vi "SetAllOccurrences.vi"(0 "occurrences":refnum<k4>[](array[refnum])) -> ()   [LabVIEW 2019, in "MessengerM.lvlib" / "SubChannelCPU.lvclass"]
uses:
  SubChannelCPU.lvclass
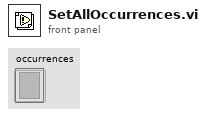
[diagram p1: front panel]
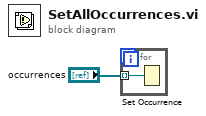
[diagram p0: block diagram]
diagram:
  n1 = for {
    tunnel: "occurrences" -> [w2] mode=indexing
    n2 = Set Occurrence(w2) -> ()
  }
